vi "Example Interrupt.vi"() -> ()   [LabVIEW 2013]
uses:
  C:/tf/play/labview/Tinkerforge.dll
panel:
  out "value mask":bool[](array[boolean])
  out "interrupt mask":bool[](array[boolean])
  in  "stop":bool
  in  "uid":string="hf4"
  in  "port":i32=4223
  in  "host":string="localhost"
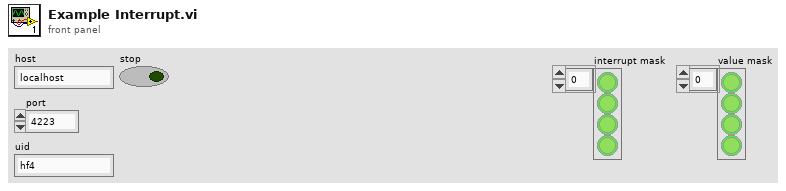
[diagram p1: front panel]
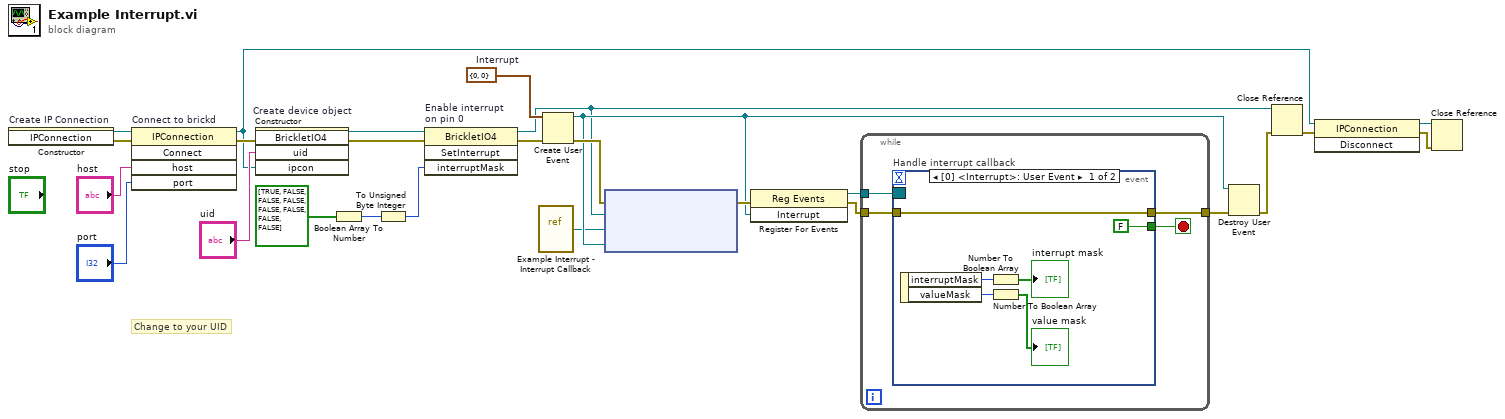
[diagram p0: block diagram]
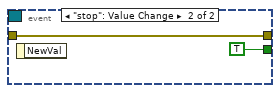
[diagram p2: hidden frame]
diagram:
  w10 = cluster{"interruptMask":u8, "valueMask":u8} {"interruptMask"=0, "valueMask"=0}  # Interrupt
  # "Change to your UID"
  n1 = constructor on="Create IP Connection" class="IPConnection"() -> (reference out=w26:refnum<k24>, error out=w5:errorcluster)  [unwired: 3 in, 1 out]
  n2 = invoke on="Connect to brickd" class="IPConnection" method="Connect"(reference=w26, error in=w5, "host"="host", "port"="port") -> (reference out=w19:refnum<k24>, error out=w22:errorcluster)  [unwired: 1 in, 3 out]
  n3 = constructor on="Create device object" class="BrickletIO4"(error in=w22, "uid"="uid", "ipcon"=w19) -> (reference out=w7:refnum<k24>, error out=w9:errorcluster)  [unwired: 2 in, 3 out]
  n4 = Boolean Array To Number(Boolean array=bool[] [TRUE, FALSE, FALSE, FALSE, FALSE, FALSE, FALSE, FALSE]) -> (number=w3:u32)
  n5 = To Unsigned Byte Integer(number=w3) -> (unsigned 8bit integer=w2:u8)
  n6 = invoke on="Enable interrupt\non pin 0" class="BrickletIO4" method="SetInterrupt"(reference=w7, error in=w9, "interruptMask"=w2) -> (reference out=w6:refnum<k24>, error out=w8:errorcluster)  [unwired: 1 in, 2 out]
  n7 = vi-ref "Example Interrupt - Interrupt Callback.vi"() -> ("vi reference"=w1:refnum<vi>)
  n8 = Create User Event(user event datatype=w10, error in=w8) -> (user event=w12:refnum<user-event>, error out=w17:errorcluster)
  n9 = node ("Register Event Callback")(w17, w6, w1, w12) -> (w16:errorcluster)  [unwired: 1 in, 1 out]
  n10 = register-events(error in=w16, w12) -> (reference out=w15:refnum<event-registration>, error out=w13:errorcluster)  [unwired: 1 in]
  n11 = while {
    tunnel: w15 -> [w30]
    tunnel: [w29] -> w14
    tunnel: w13 -> [w28]
    stop <- w27 stop-if-true
    n12 = event "Handle interrupt callback" shown="[0] <Interrupt>: User Event" {
      selector: w30 -> [_ _]
      dyn-events: _ -> [_ _]
      timeout: _ -> [_ _]
      tunnel: [w36 w37] -> w29
      tunnel: w28 -> [w36 w37]
      tunnel: [FALSE TRUE] -> w27
      event User Event {
        n13 = event-data() -> ("interruptMask"=w31:u8, "valueMask"=w34:u8)  [unwired: 1 in]
        n14 = Number To Boolean Array(number=w31) -> (Boolean array=→"interrupt mask":bool[])
        n15 = Number To Boolean Array(number=w34) -> (Boolean array=→"value mask":bool[])
      }
      event "stop": Value Change {
        n16 = event-data() -> ()  [unwired: 1 in, 1 out]
      }
    }
  }
  n17 = Destroy User Event(user event=w12, error in=w14) -> (error out=w11:errorcluster)
  n18 = Close Reference(reference=w6, error in (no error)=w11) -> (error out=w21:errorcluster)
  n19 = invoke class="IPConnection" method="Disconnect"(reference=w19, error in=w21) -> (reference out=w18:refnum<k24>, error out=w20:errorcluster)  [unwired: 1 in, 1 out]
  n20 = Close Reference(reference=w18, error in (no error)=w20) -> ()  [unwired: 1 out]
